vi "update_card_FB.vi"(8 "error in (no error)":errorcluster, 10 "Card":bool, 11 "Card_detection in":refnum<class "Card_detection.lvclass">) -> (0 "error out":errorcluster, 3 "Card_detection out":refnum<class "Card_detection.lvclass">)   [LabVIEW 2025, in "User_Console-ATM.lvlib" / "Card_detection.lvclass"]
uses:
  Card_detection.lvclass
  Card_detection.lvclass/Card_detection.ctl
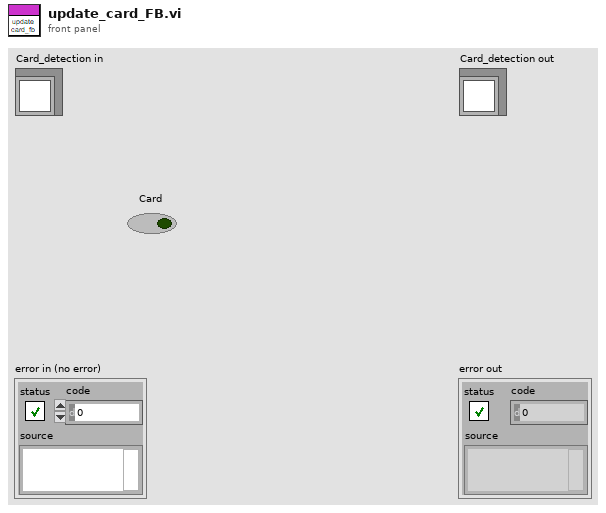
[diagram p1: front panel]
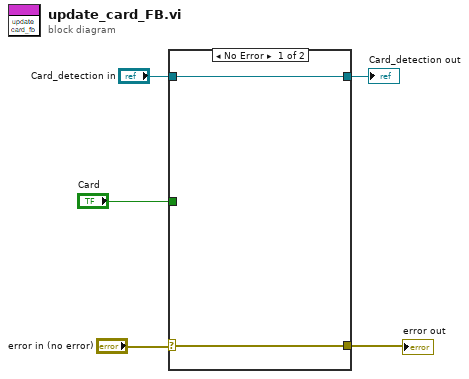
[diagram p0: block diagram]
diagram:
  n1 = case shown="No Error" "error in (no error)" {
    selector: "error in (no error)" -> [w7 w8]
    tunnel: [w7 w8] -> w4
    tunnel: "Card_detection in" -> [w6 w9]
    tunnel: [w6 w9] -> w2
    tunnel: "Card" -> [_ _]
    frame No Error {
    }
    frame Error {
    }
  }
  "error out" <- w4
  "Card_detection out" <- w2
